vi "set_multiramp_soak_profile_segment_soak_value.vi"(8 "error in (no error)":errorcluster, 9 "Soak value (C)":dbl, 10 "Segment number":u8 max=15, 11 "VISA Refnum in":refnum<visa-resource-name>) -> (0 "error out":errorcluster, 3 "VISA Refnum out":refnum<visa-resource-name>)   [LabVIEW 2018]
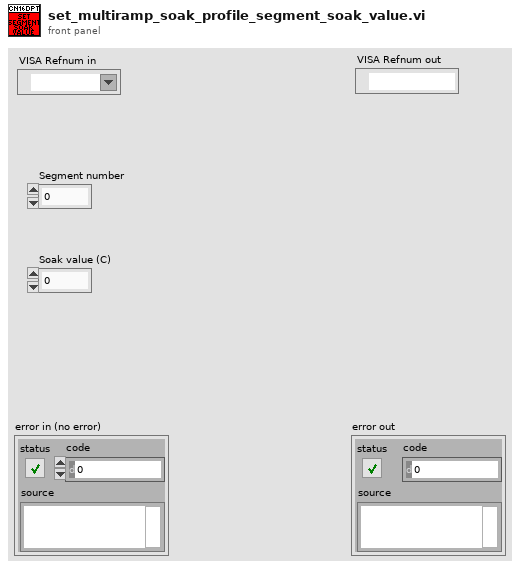
[diagram p1: front panel]
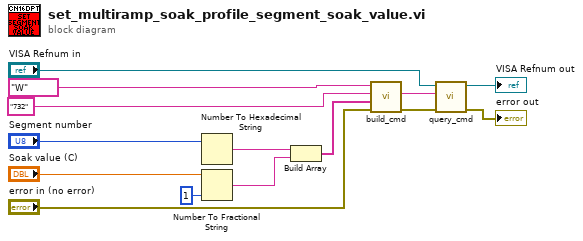
[diagram p0: block diagram]
diagram:
  n1 = Number To Hexadecimal String(2:"Segment number") -> (0:w4:string)  [unwired: 1 in]
  n2 = Number To Fractional String(number="Soak value (C)", precision (6)=i16 1) -> (F-format string=w3:string)  [unwired: 2 in]
  n3 = Build Array(w4, w3) -> (w6:string[])
  n4 = call "build_cmd.vi"("error in (no error)"="error in (no error)", "Parameter list"=w6, "Command ID"="732", "Command class"="W") -> ("error out"=w9:errorcluster, "Command"=w8:string)  [unwired: 6 in]
  n5 = call "query_cmd.vi"("error in (no error)"=w9, "Command"=w8, "VISA resource name"="VISA Refnum in") -> ("error out"=→"error out":errorcluster, "VISA resource name out"=→"VISA Refnum out":refnum<visa-resource-name>)  [unwired: 6 in, 1 out]
